vi "Waveplatecontrol_stepscan.vi"() -> ()   [LabVIEW 2015]
uses:
  subvi/Newport ESP301/Newport ESP301.lvlib
  <vilib>/DAQmx/create/channels.llb/DAQmx Create Channel (AO-Voltage-Basic).vi
  <vilib>/DAQmx/write.llb/DAQmx Write (Analog DBL 1Chan 1Samp).vi
panel:
  in  "p1 [deg] 3":dbl
  in  "p1 [deg] 2":dbl
  in  "Numeric":i32=10
  in  "Stepsize":dbl
  in  "ms2wait":u32
  in  "Boolean":bool
  out "a":waveform(dbl)(graph)={"t0"=timestamp(3620209335.8073797 s since 1904-01-01), "dt"=1.0, "Y"=[nan]}
  out "Waveform Chart":dbl(graph)=5.25341140860948
  out "x*y":dbl=nan
  in  "physical channels":tag="Dev3/ao1"
  out "DAC error":errorcluster
  out "ESP error":errorcluster={"status"=TRUE, "code"=-1073807343, "source"="VISA Open in Newport ESP301.lvlib:Initialize.vi->main002.vi"}
  out "run?":bool
  in  "set_vel":bool
  in  "velocity [fs/s]":dbl=667.128190396304
  in  "vel_mm":dbl caption="velocity [deg/s]"
  out "meas. velocity":dbl=nan
  in  "stop":bool
  out "output voltage":dbl=nan
  in  "start":bool
  in  "go2p1":bool
  out "position [deg]":dbl=nan
  in  "p2 [deg]":dbl=2.0
  in  "p1 [deg]":dbl
  in  "interpolate output":bool
  in  "Delta2 [deg]":dbl=6671.281903963041
  in  "Delta1 [deg]":dbl=-6671.281903963041
  in  "Reference [deg]":dbl=1.0
  in  "Axis (1)":i32=2 min=1 max=3
  in  "Serial Link (RS232)":enum16{"RS232", "USB"}(ring)
  in  "VISA resource name":refnum<visa-resource-name>="COM9"
  in  "main_close":bool
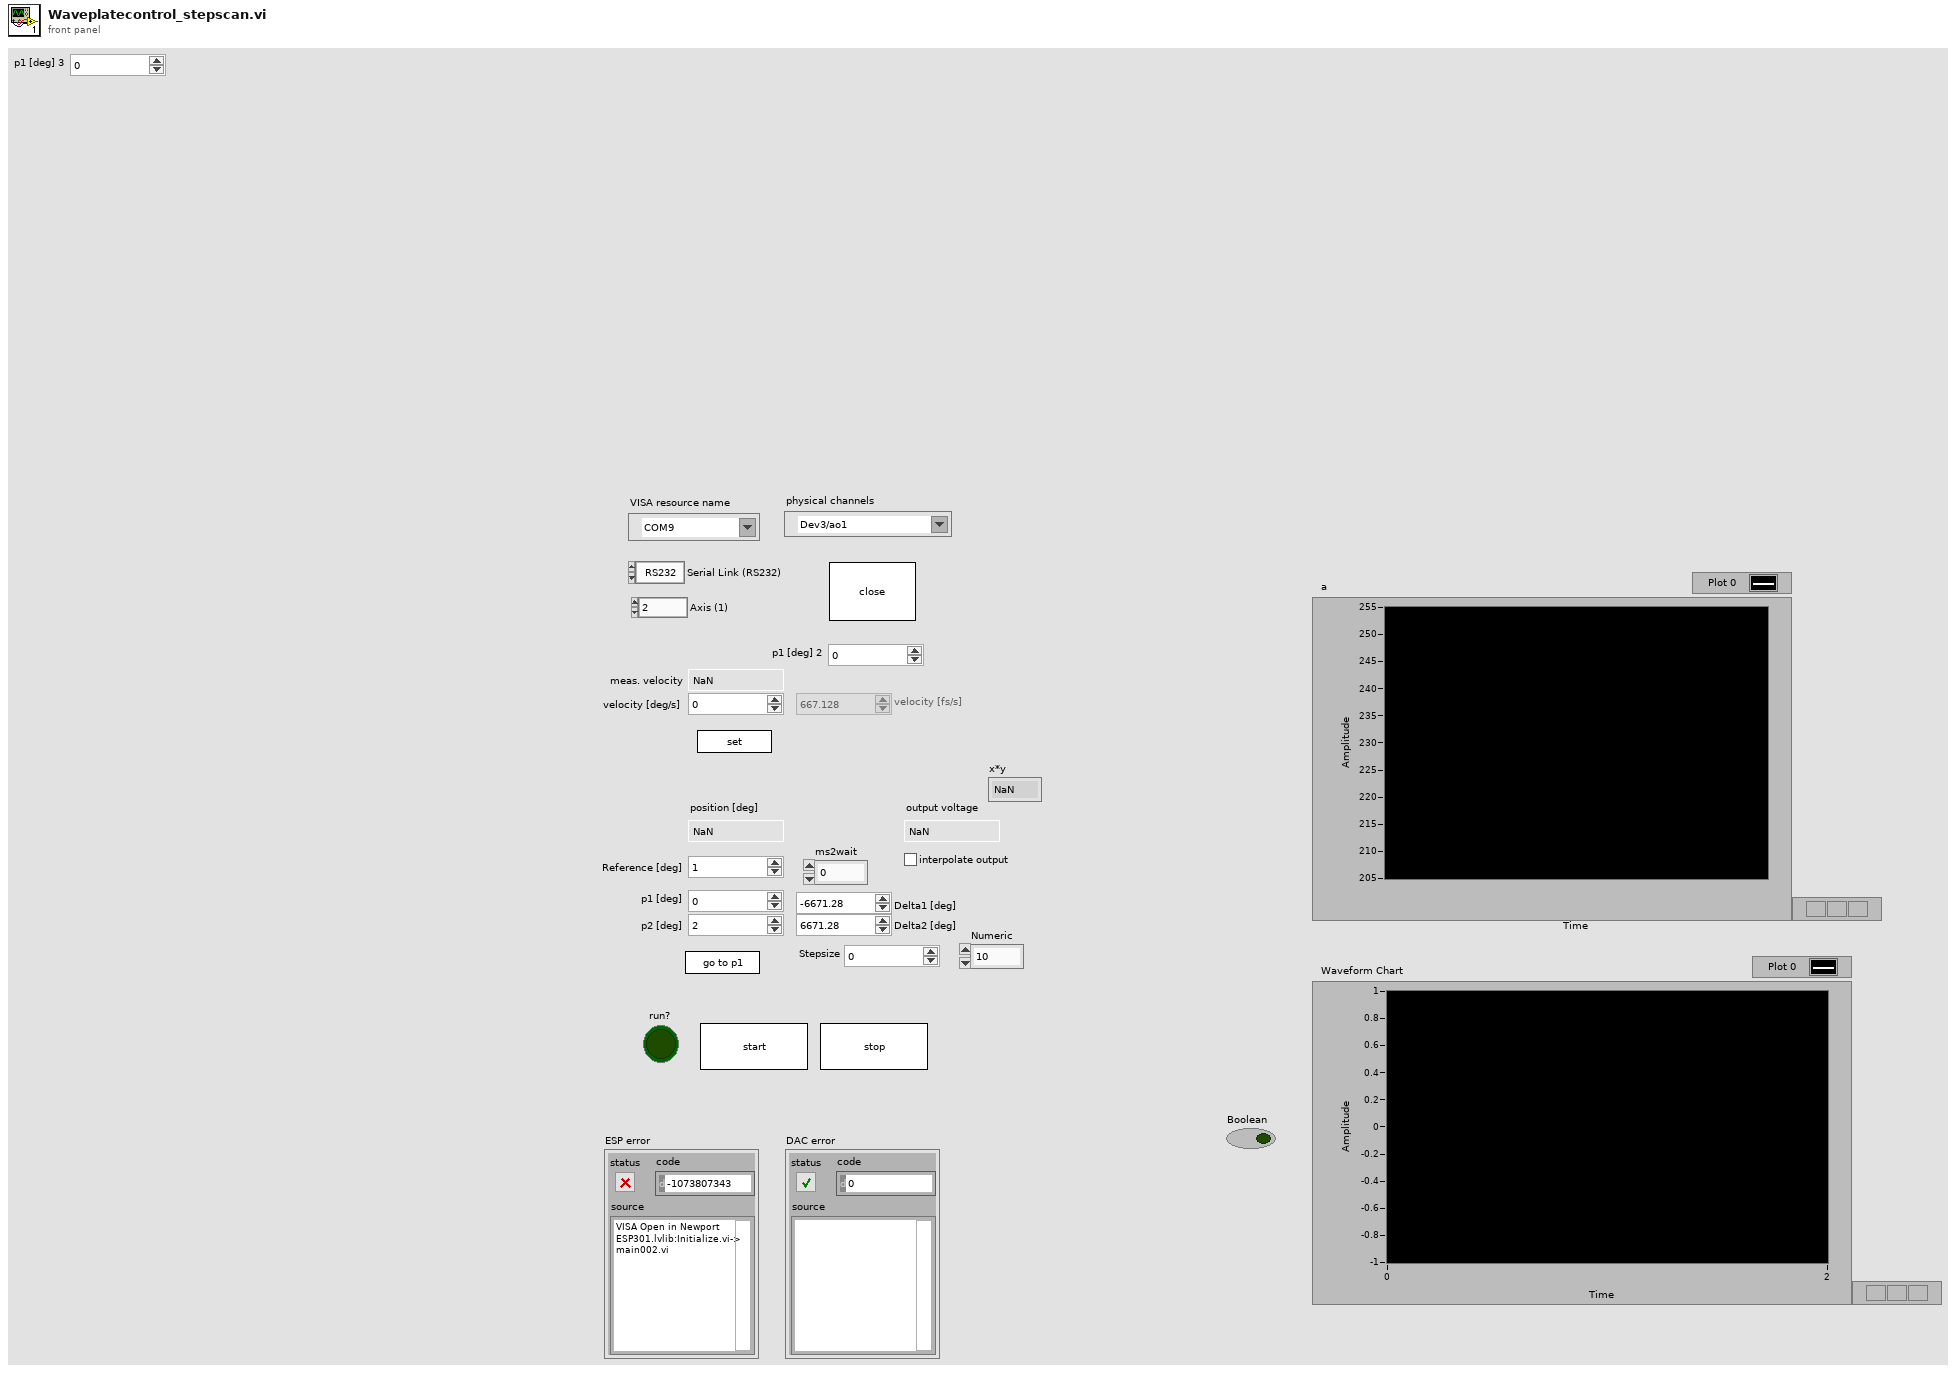
[diagram p1: front panel]
types:
  T1 = cluster{"dev1_data":refnum<queue>, "dev2_data":refnum<queue>}
  T2 = cluster{"dev1_cmd":refnum<queue>, "dev2_cmd":refnum<queue>}
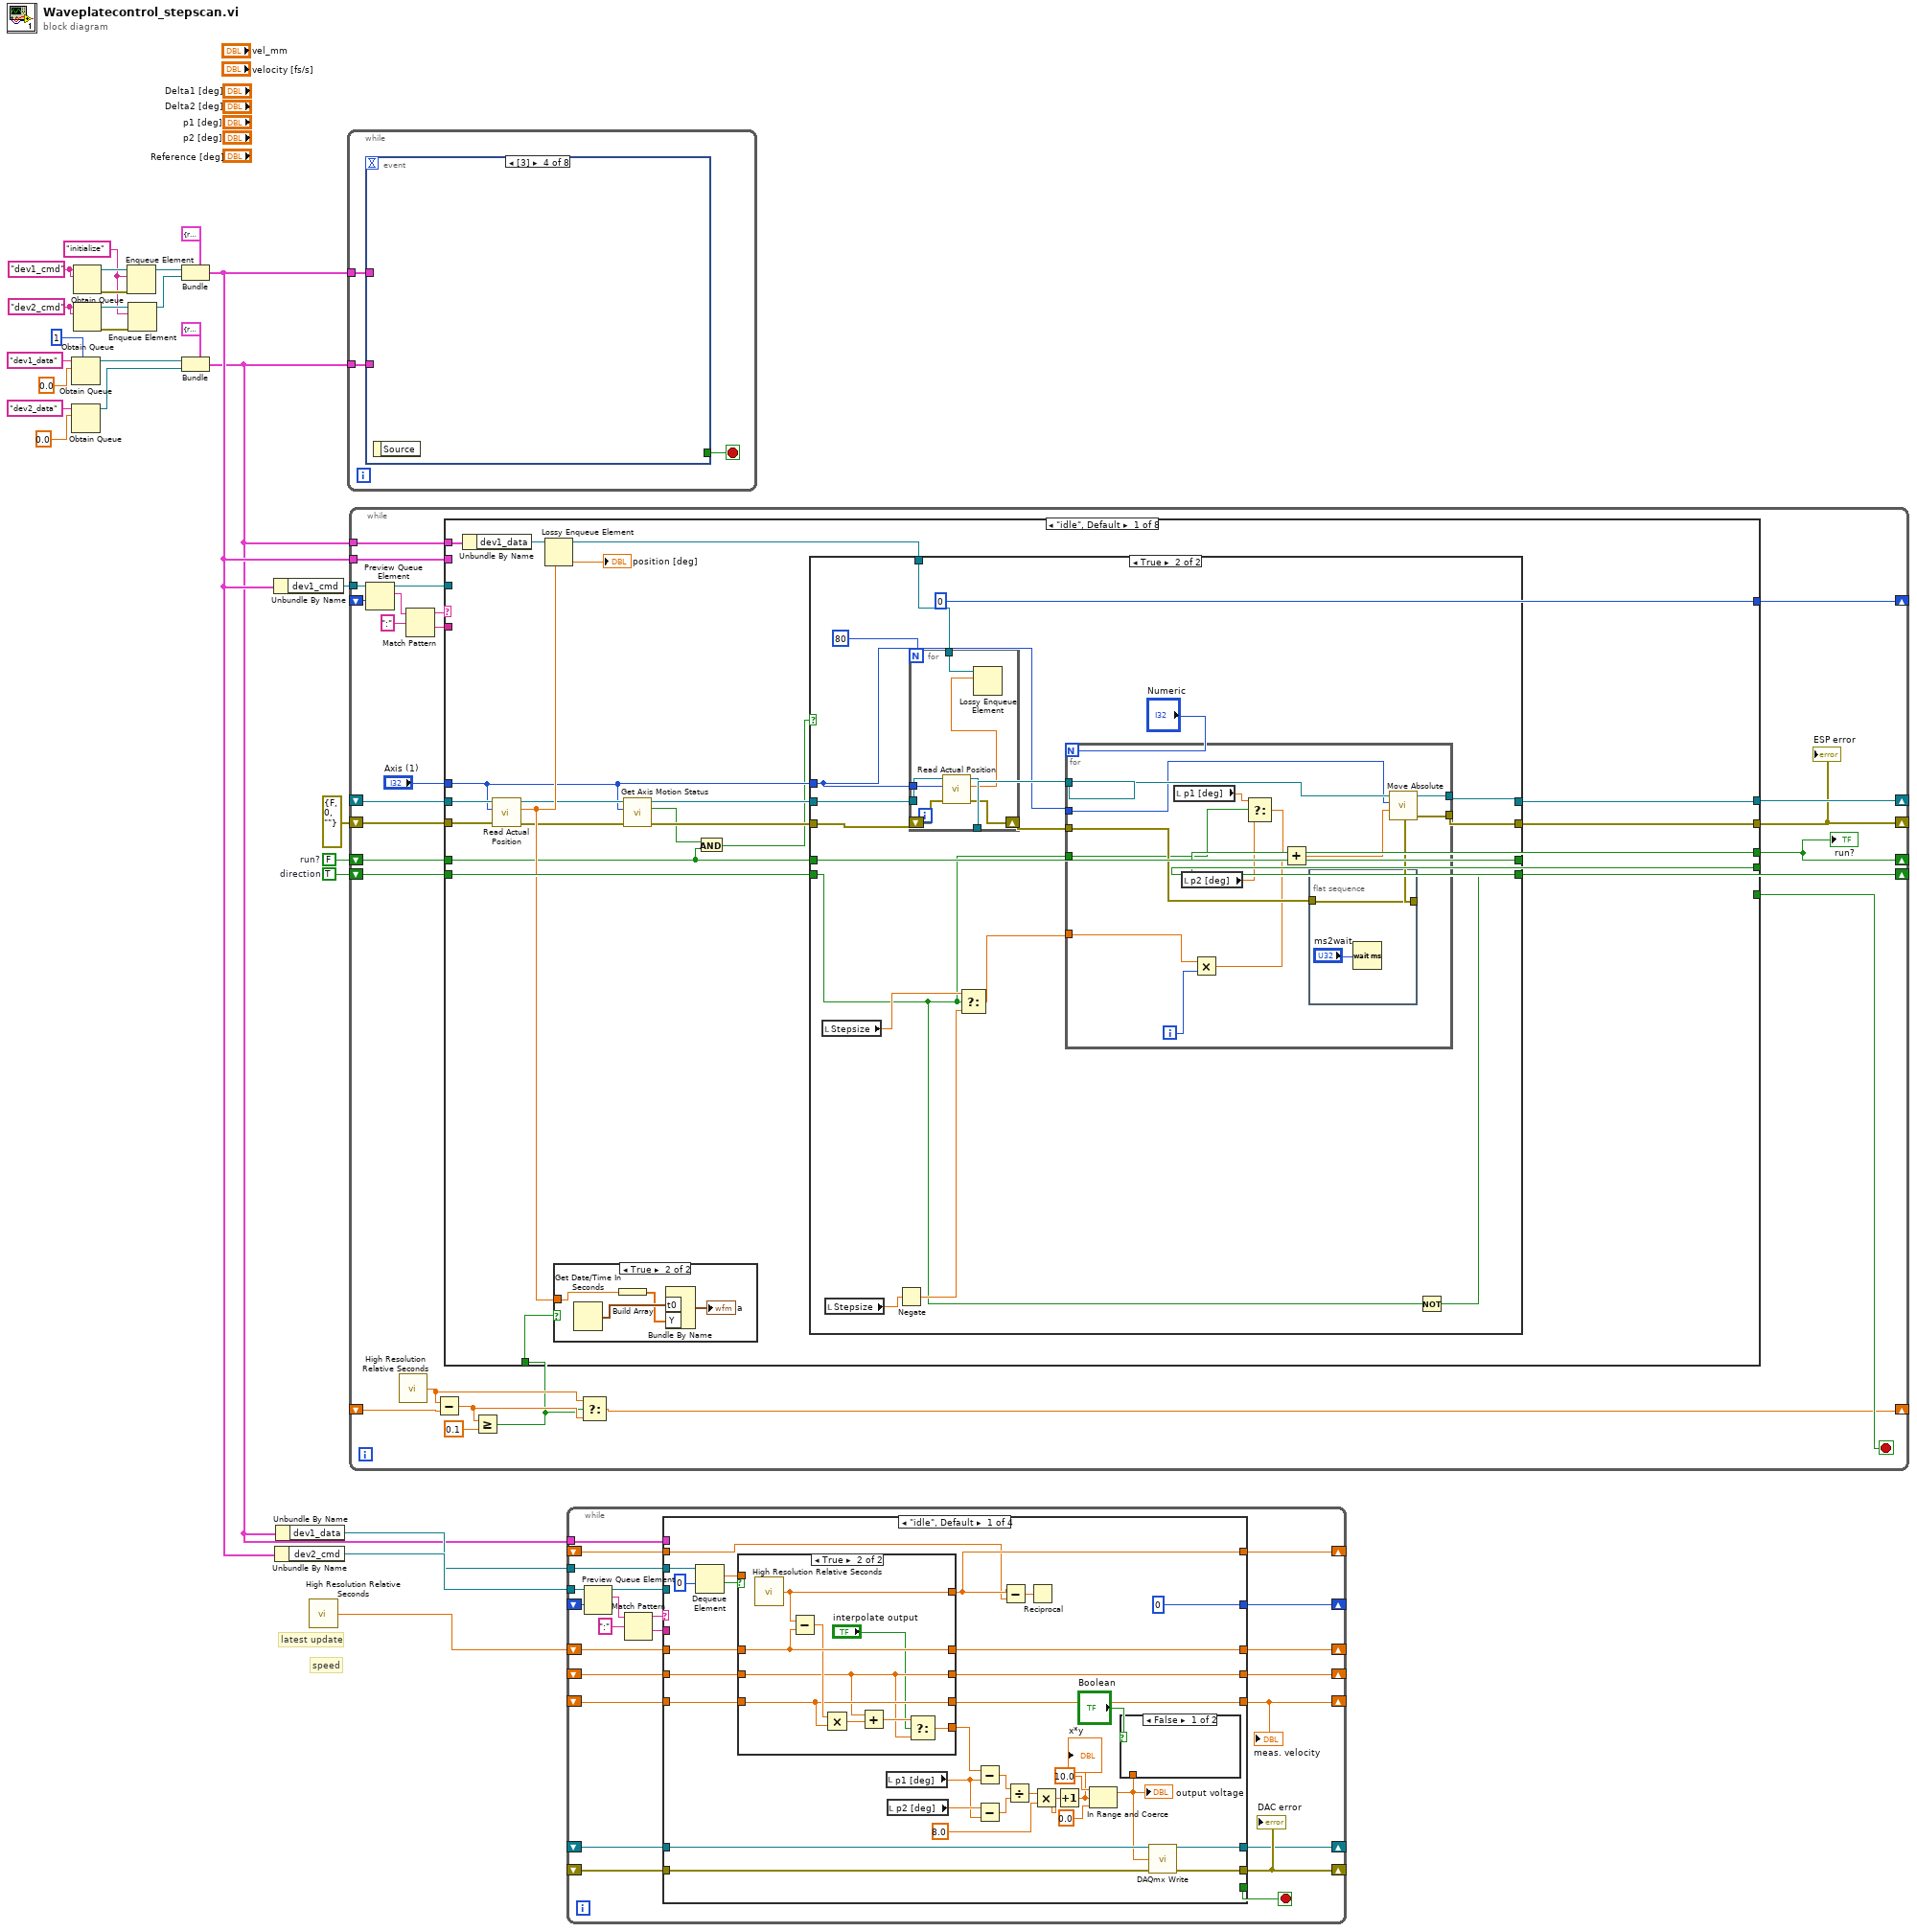
[diagram p0: block diagram]
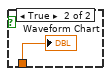
[diagram p2: hidden frame]
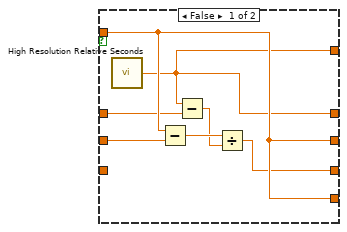
[diagram p3: hidden frame]
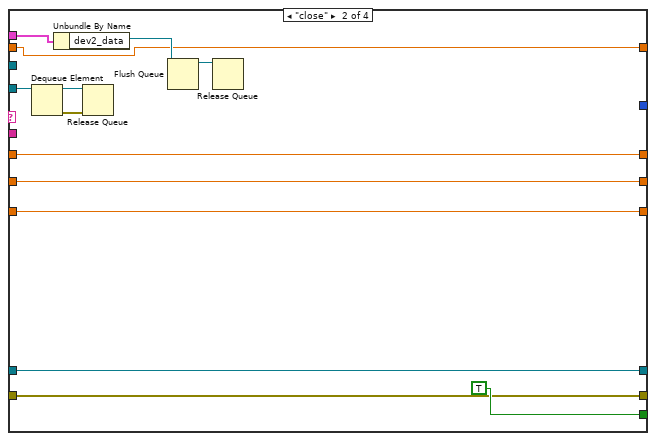
[diagram p4: hidden frame]
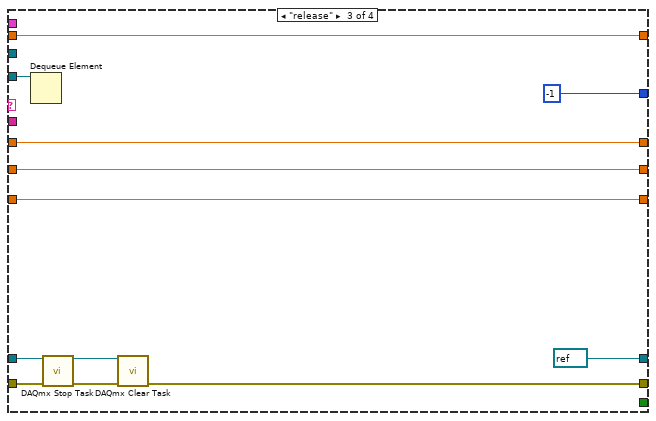
[diagram p5: hidden frame]
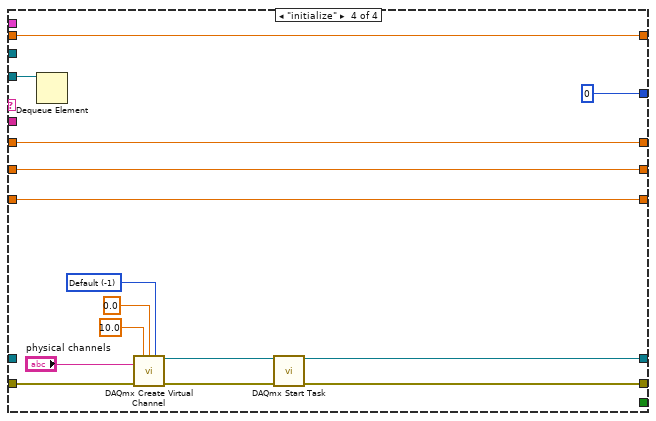
[diagram p6: hidden frame]
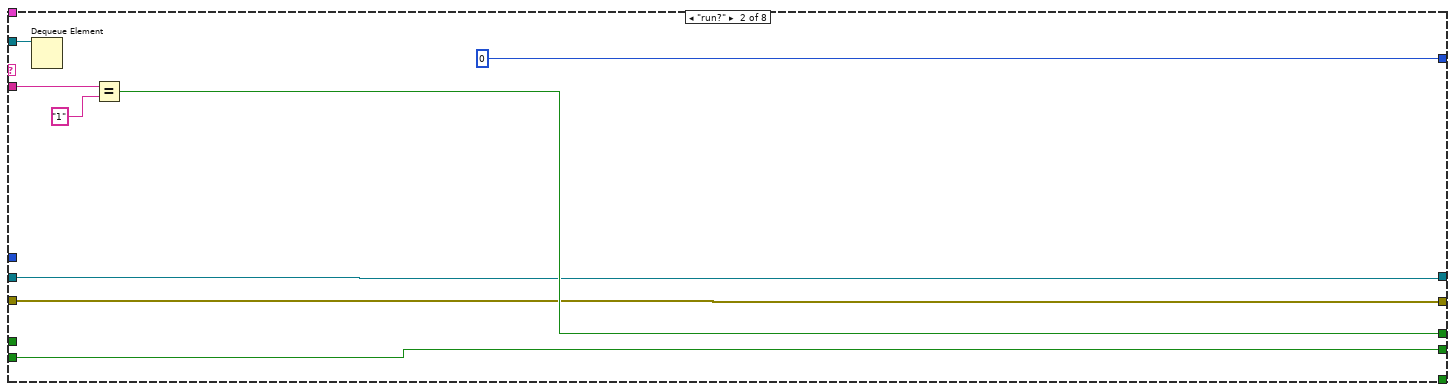
[diagram p9: hidden frame]
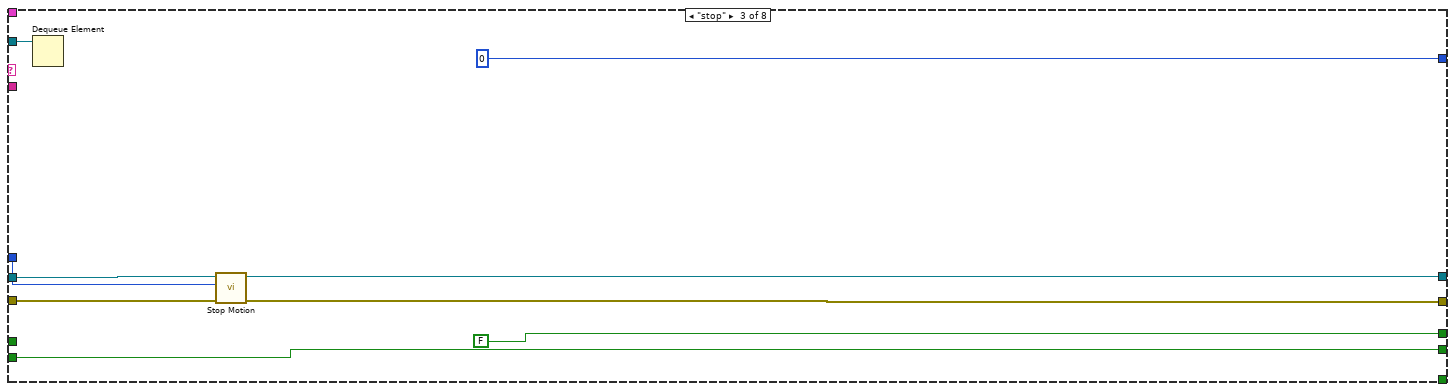
[diagram p10: hidden frame]
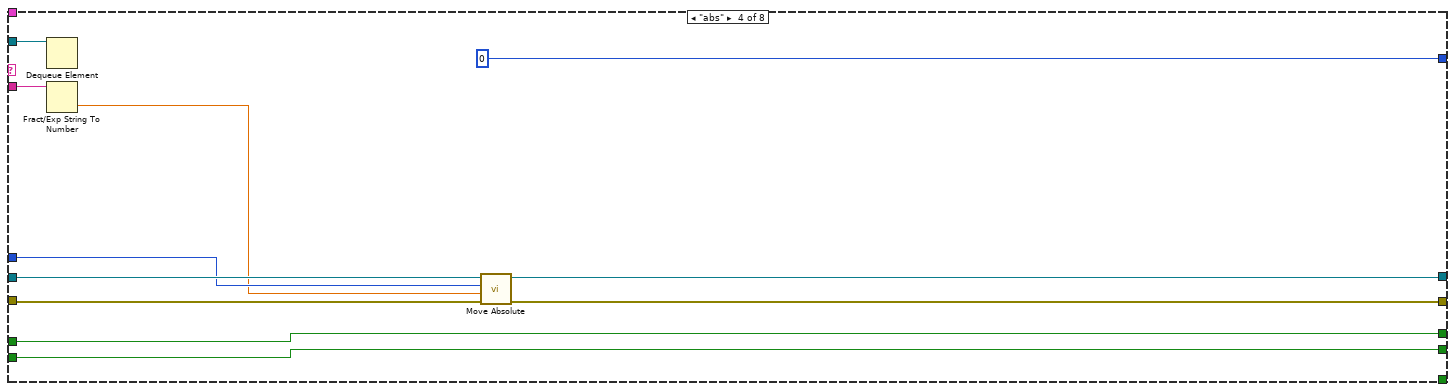
[diagram p11: hidden frame]
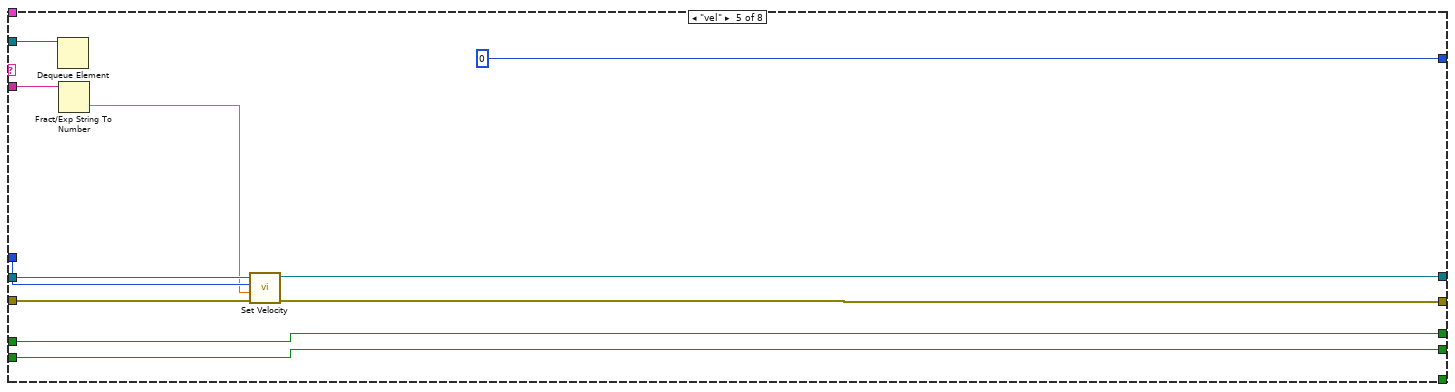
[diagram p12: hidden frame]
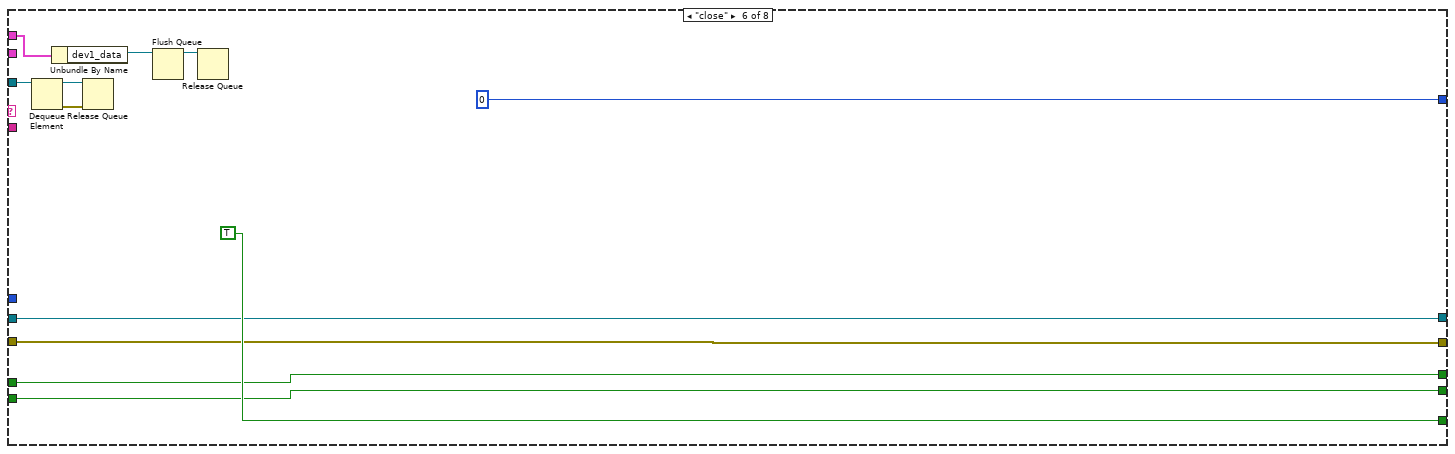
[diagram p13: hidden frame]
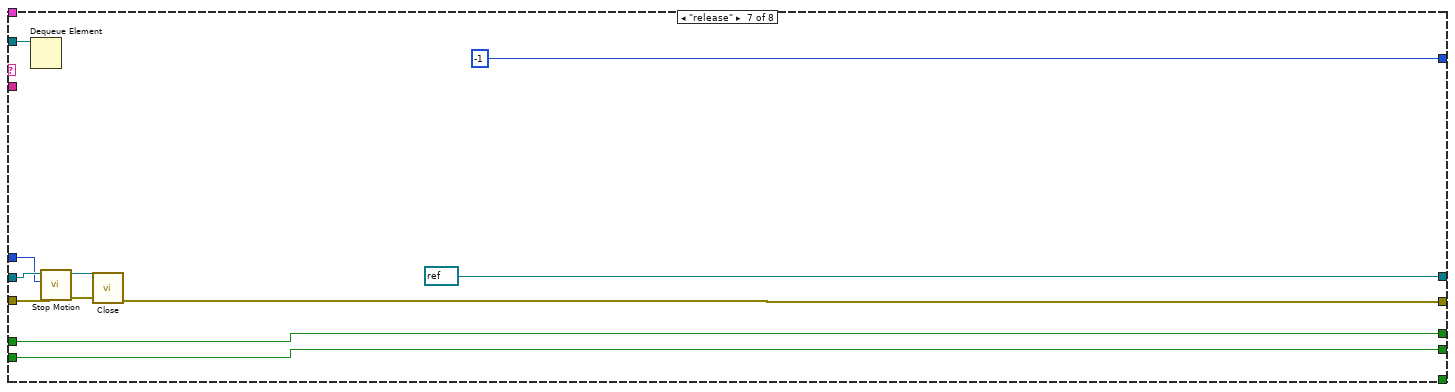
[diagram p14: hidden frame]
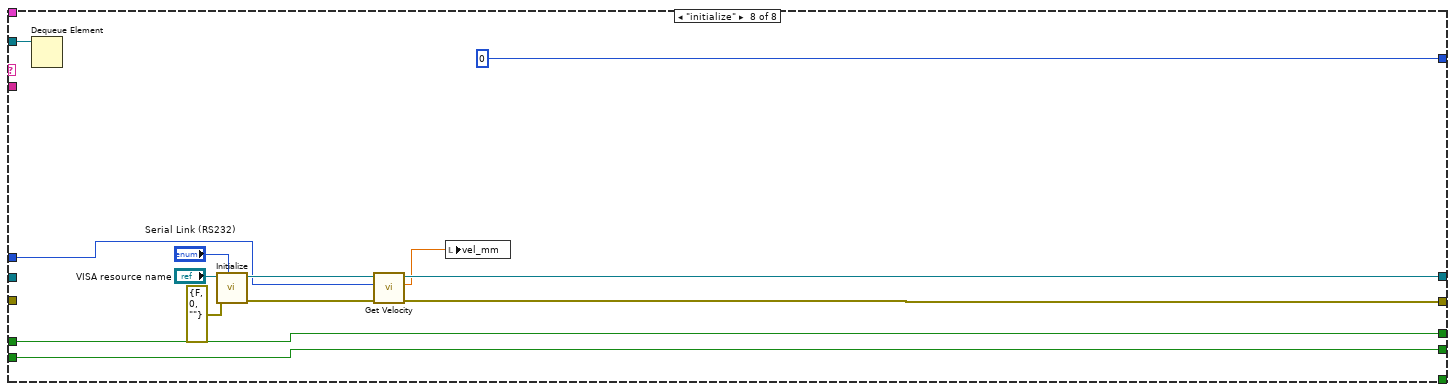
[diagram p15: hidden frame]
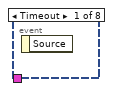
[diagram p16: hidden frame]
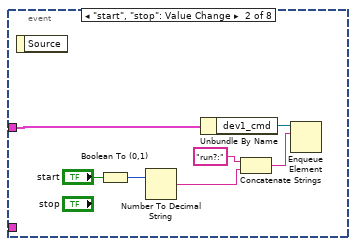
[diagram p17: hidden frame]
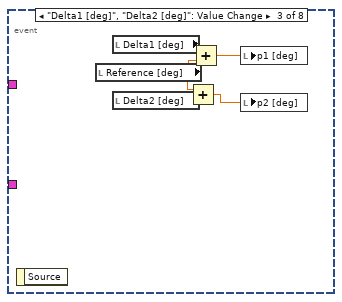
[diagram p18: hidden frame]
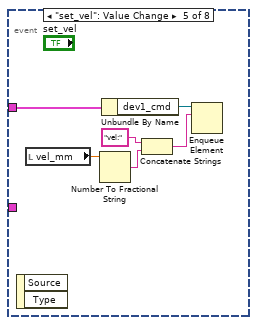
[diagram p19: hidden frame]
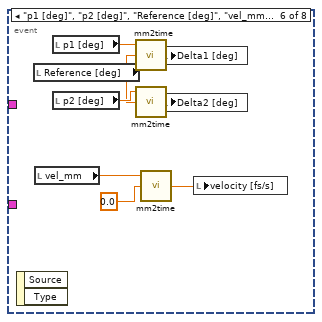
[diagram p20: hidden frame]
diagram:
  w1 = TRUE  # direction
  w4 = FALSE  # run?
  w15 = "dev2_cmd" ("name (unnamed)")
  w21 = "initialize" ("element")
  w16 = "dev1_cmd" ("name (unnamed)")
  # "speed"
  # "latest update"
  n1 = Obtain Queue(max queue size (-1, unlimited)=1, name (unnamed)="dev1_data", element data type=0.0) -> (queue out=w12:refnum<queue>)  [unwired: 2 in, 2 out]
  n2 = Obtain Queue(name (unnamed)="dev2_data", element data type=0.0) -> (queue out=w11:refnum<queue>)  [unwired: 3 in, 2 out]
  n3 = Obtain Queue(name (unnamed)=w16, element data type=w16) -> (queue out=w27:refnum<queue>, error out=w26:errorcluster)  [unwired: 3 in, 1 out]
  n4 = Obtain Queue(name (unnamed)=w15, element data type=w15) -> (queue out=w22:refnum<queue>, error out=w23:errorcluster)  [unwired: 3 in, 1 out]
  n5 = Enqueue Element(queue=w27, element=w21, error in (no error)=w26) -> (queue out=w24:refnum<queue>)  [unwired: 1 in, 2 out]
  n6 = Enqueue Element(queue=w22, element=w21, error in (no error)=w23) -> (queue out=w20:refnum<queue>)  [unwired: 1 in, 2 out]
  n7 = Bundle(cluster=T2 {"dev1_cmd"=refnum, "dev2_cmd"=refnum}, "dev1_cmd"=w24, "dev2_cmd"=w20) -> (w8:T2)
  n8 = Bundle(cluster=T1 {"dev1_data"=refnum, "dev2_data"=refnum}, "dev1_data"=w12, "dev2_data"=w11) -> (w2:T1)
  n9 = Unbundle By Name(w8) -> ("dev1_cmd"=w17:refnum<queue>)
  n10 = Unbundle By Name(w8) -> ("dev2_cmd"=w7:refnum<queue>)
  n11 = Unbundle By Name(w2) -> ("dev1_data"=w6:refnum<queue>)
  n12 = call <vilib>:"High Resolution Relative Seconds.vi"() -> ("relative seconds"=w5:dbl)
  n13 = while {
    tunnel: w8 -> [w30]
    tunnel: w2 -> [w29]
    stop <- w28 stop-if-true
    n14 = event shown="[3]" {
      selector: _ -> [_ _ _ _ _ _ _ _]
      dyn-events: _ -> [_ _ _ _ _ _ _ _]
      timeout: _ -> [_ _ _ _ _ _ _ _]
      tunnel: w30 -> [_ w34 _ _ w44 _ w62 w65]
      tunnel: w29 -> [_ _ _ _ _ _ _ _]
      tunnel: [_ _ _ _ _ _ _ TRUE] -> w28
      event Timeout {
        n15 = event-data() -> ()  [unwired: 1 in, 1 out]
      }
      event "start", "stop": Value Change {
        n16 = event-data() -> ()  [unwired: 1 in, 1 out]
        n17 = Boolean To (0,1)(Boolean="start") -> (0, 1=w32:i16)
        n18 = Number To Decimal String(number=w32) -> (decimal integer string=w31:string)  [unwired: 1 in]
        n19 = Unbundle By Name(w34) -> ("dev1_cmd"=w37:refnum<queue>)
        n20 = Concatenate Strings("run?:" ("string"), w31) -> (w36:string)
        n21 = Enqueue Element(queue=w37, element=w36) -> ()  [unwired: 2 in, 3 out]
      }
      event "Delta1 [deg]", "Delta2 [deg]": Value Change {
        n22 = event-data() -> ()  [unwired: 1 in, 1 out]
        n23 = local read "Reference [deg]"() -> (w40:dbl)
        n24 = local read "Delta1 [deg]"() -> (w42:dbl)
        n25 = local read "Delta2 [deg]"() -> (w41:dbl)
        n26 = Add(x=w40, y=w41) -> (x+y=w38:dbl)
        n27 = Add(x=w42, y=w40) -> (x+y=w39:dbl)
        n28 = local write "p1 [deg]"(w39) -> ()
        n29 = local write "p2 [deg]"(w38) -> ()
      }
      event #3 (no event record) {
        n30 = event-data() -> ()  [unwired: 1 in, 1 out]
        n31 = local read "p1 [deg] 3"() -> ()  [unwired: 1 out]
      }
      event "set_vel": Value Change {
        n32 = event-data() -> ()  [unwired: 1 in, 2 out]
        n33 = local read "vel_mm"() -> (w43:dbl)
        n34 = Number To Fractional String(number=w43) -> (F-format string=w47:string)  [unwired: 3 in]
        n35 = Unbundle By Name(w44) -> ("dev1_cmd"=w48:refnum<queue>)
        n36 = Concatenate Strings("vel:" ("string"), w47) -> (w46:string)
        n37 = Enqueue Element(queue=w48, element=w46) -> ()  [unwired: 2 in, 3 out]
      }
      event "p1 [deg]", "p2 [deg]", "Reference [deg]", "vel_mm": Value Change {
        n38 = event-data() -> ()  [unwired: 1 in, 2 out]
        n39 = local read "Reference [deg]"() -> (w54:dbl)
        n40 = local read "vel_mm"() -> (w51:dbl)
        n41 = local read "p1 [deg]"() -> (w55:dbl)
        n42 = local read "p2 [deg]"() -> (w56:dbl)
        n43 = call "mm2time.vi"("Offset (mm)"=w54, "distance (mm)"=w55) -> ("time in fs"=w52:dbl)  [unwired: 1 in]
        n44 = call "mm2time.vi"("Offset (mm)"=w54, "distance (mm)"=w56) -> ("time in fs"=w53:dbl)  [unwired: 1 in]
        n45 = call "mm2time.vi"("Offset (mm)"=0.0, "distance (mm)"=w51) -> ("time in fs"=w50:dbl)  [unwired: 1 in]
        n46 = local write "Delta1 [deg]"(w52) -> ()
        n47 = local write "Delta2 [deg]"(w53) -> ()
        n48 = local write "velocity [fs/s]"(w50) -> ()
      }
      event "go2p1": Value Change {
        n49 = event-data() -> ()  [unwired: 1 in, 2 out]
        n50 = local read "p1 [deg]"() -> (w57:dbl)
        n51 = Number To Fractional String(number=w57) -> (F-format string=w60:string)  [unwired: 3 in]
        n52 = Unbundle By Name(w62) -> ("dev1_cmd"=w61:refnum<queue>)
        n53 = Concatenate Strings("abs:" ("string"), w60) -> (w58:string)
        n54 = Enqueue Element(queue=w61, element=w58) -> ()  [unwired: 2 in, 3 out]
      }
      event "main_close": Value Change {
        n55 = event-data() -> ()  [unwired: 1 in, 1 out]
        n56 = Cluster To Array(cluster=w65) -> (array=w64:refnum<queue>[])
        n57 = for {
          tunnel: w64 -> [w70] mode=indexing
          n58 = Flush Queue(queue=w70) -> (queue out=w66:refnum<queue>)  [unwired: 1 in, 2 out]
          n59 = Enqueue Element(queue=w66, element="release") -> (queue out=w68:refnum<queue>)  [unwired: 2 in, 2 out]
          n60 = Enqueue Element(queue=w68, element="close") -> ()  [unwired: 2 in, 3 out]
        }
      }
    }
  }
  n61 = while {
    tunnel: w8 -> [w91]
    tunnel: w17 -> [w96]
    tunnel: w2 -> [w88]
    shift-right: [w86] -> _
    shift-left: _ -> [w87]
    shift-right: [w85] -> _
    shift-left: _ -> [w82]
    shift-right: [w84] -> _
    shift-left: errorcluster {"status"=FALSE, "code"=0, "source"=""} ("error out") -> [w83]
    shift-right: [w79] -> _
    shift-left: w4 -> [w80]
    shift-right: [w77] -> _
    shift-left: w1 -> [w78]
    shift-right: [w71] -> _
    shift-left: _ -> [w76]
    stop <- w89 stop-if-true
    n62 = Preview Queue Element(queue=w96, timeout in ms (-1)=w87) -> (queue out=w90:refnum<queue>, element=w95:string)  [unwired: 1 in, 2 out]
    n63 = call <vilib>:"High Resolution Relative Seconds.vi"() -> ("relative seconds"=w73:dbl)
    n64 = Match Pattern(string=w95, regular expression=":") -> (before substring=w93:string, after substring=w92:string)  [unwired: 1 in, 2 out]
    n65 = Subtract(x=w73, y=w76) -> (x-y=w74:dbl)
    n66 = Greater Or Equal?(x=w74, y=0.1) -> (x >= y?=w72:bool)
    n67 = case shown="\"idle\", Default" w93 {
      tunnel: w92 -> [_ w173 _ w192 w199 _ _ _]
      tunnel: w91 -> [_ _ _ _ _ _ _ _]
      tunnel: w90 -> [_ w171 w175 w193 w197 w216 w226 w236]
      tunnel: [_ _ _ _ _ TRUE _ _] -> w89
      tunnel: w88 -> [w116 _ _ _ _ w208 _ _]
      tunnel: [0 0 0 0 0 0 -1 0] -> w86
      tunnel: [w114 w166 w180 w189 w204 w212 refnum<visa-resource-name> refnum ("VISA resource name out") w232] -> w85
      tunnel: [w113 w167 w179 w188 w203 w211 w225 w231] -> w84
      tunnel: w83 -> [w111 w167 w181 w190 w202 w211 w221 _]
      tunnel: w82 -> [w112 w166 w182 w191 w201 w212 w218 _]
      tunnel: "Axis (1)" -> [w100 _ w178 w187 w200 _ w217 w233]
      tunnel: w80 -> [w98 _ _ w184 w195 w209 w223 w237]
      tunnel: [w108 w169 FALSE ("run?") w184 w195 w209 w223 w237] -> w79
      tunnel: w78 -> [w109 w168 w174 w183 w194 w205 w222 w228]
      tunnel: [w110 w168 w174 w183 w194 w205 w222 w228] -> w77
      tunnel: w72 -> [w107 _ _ _ _ _ _ _]
      frame "idle", Default {
        n68 = Unbundle By Name(w116) -> ("dev1_data"=w115:refnum<queue>)
        n69 = call "Read Actual Position.vi"("error in (no error)"=w111, "Axis (1)"=w100, "VISA resource name"=w112) -> ("error out"=w103:errorcluster, "Position (units)"=w105:dbl, "VISA resource name out"=w104:refnum<visa-resource-name>)  [unwired: 2 in]
        "position [deg]" <- w105
        n70 = Lossy Enqueue Element(queue=w115, element=w105) -> (queue out=w106:refnum<queue>)  [unwired: 1 in, 3 out]
        n71 = case shown="True" w107 {
          tunnel: w105 -> [_ w121]
          frame False {
          }
          frame True {
            n72 = Get Date/Time In Seconds() -> (seconds since 1Jan1904=w120:timestamp)
            n73 = Build Array(w121) -> (w119:dbl[])
            n74 = Bundle By Name("t0"=w120, "Y"=w119) -> (→"a":waveform(dbl))  [unwired: 1 in]
          }
        }
        n75 = call "Get Axis Motion Status.vi"("error in (no error)"=w103, "Axis (1)"=w100, "VISA resource name"=w104) -> ("error out"=w101:errorcluster, "Motion Done"=w99:bool, "VISA resource name out"=w102:refnum<visa-resource-name>)  [unwired: 2 in]
        n76 = And(x=w99, y=w98) -> (x .and. y?=w97:bool)
        n77 = case shown="True" w97 {
          tunnel: w102 -> [w125 w138]
          tunnel: w101 -> [w124 w139]
          tunnel: [w125 w134] -> w114
          tunnel: [w124 w135] -> w113
          tunnel: w100 -> [_ w132]
          tunnel: [w123 w137] -> w110
          tunnel: w109 -> [w123 w126]
          tunnel: w98 -> [w122 w142]
          tunnel: [w122 w142] -> w108
          tunnel: w106 -> [_ w141]
          frame False {
          }
          frame True {
            n78 = local read "Stepsize"() -> (w136:dbl)
            n79 = local read "Stepsize"() -> (w130:dbl)
            n80 = Negate(x=w130) -> (-x=w129:dbl)
            n81 = for {
              N: 80 -> [_]
              tunnel: w138 -> [w165]
              tunnel: [w164] -> w133
              shift-right: [w159] -> w131
              shift-left: w139 -> [w163]
              tunnel: w132 -> [w162]
              tunnel: w141 -> [w161]
              n82 = call "Read Actual Position.vi"("error in (no error)"=w163, "Axis (1)"=w162, "VISA resource name"=w165) -> ("error out"=w159:errorcluster, "Position (units)"=w160:dbl, "VISA resource name out"=w164:refnum<visa-resource-name>)  [unwired: 2 in]
              n83 = Lossy Enqueue Element(queue=w161, element=w160) -> ()  [unwired: 1 in, 4 out]
            }
            n84 = Select(t=w136, s=w126, f=w129) -> (s? t:f=w128:dbl)
            n85 = for {
              N: "Numeric" -> [_]
              tunnel: [w156] -> w135
              tunnel: [w155] -> w134
              tunnel: w131 -> [w152]
              tunnel: w133 -> [w154]
              tunnel: w132 -> [w153]
              tunnel: w128 -> [w149]
              tunnel: w126 -> [w144]
              i -> [w150]
              n86 = local read "p1 [deg]"() -> (w146:dbl)
              n87 = local read "p2 [deg]"() -> (w143:dbl)
              n88 = Multiply(x=w149, y=w150) -> (x*y=w148:dbl)
              n89 = Select(t=w146, s=w144, f=w143) -> (s? t:f=w145:dbl)
              n90 = Add(x=w145, y=w148) -> (x+y=w147:dbl)
              n91 = flat-sequence {
                tunnel: w152 -> [w158]
                tunnel: [w158] -> w151
                frame #0 {
                  n92 = Wait (ms)(milliseconds to wait="ms2wait") -> ()  [unwired: 1 out]
                }
              }
              n93 = call "Move Absolute.vi"("error in (no error)"=w151, "Position (0 units)"=w147, "Axis (1)"=w153, "VISA resource name"=w154) -> ("error out"=w156:errorcluster, "VISA resource name out"=w155:refnum<visa-resource-name>)  [unwired: 2 in]
              n94 = local read "p1 [deg] 2"() -> ()  [unwired: 1 out]
            }
            n95 = Not(x=w126) -> (.not. x?=w137:bool)
          }
        }
      }
      frame "run?" {
        n96 = Dequeue Element(queue=w171) -> ()  [unwired: 2 in, 4 out]
        n97 = Equal?(x=w173, y="1") -> (x = y?=w169:bool)
      }
      frame "stop" {
        n98 = Dequeue Element(queue=w175) -> ()  [unwired: 2 in, 4 out]
        n99 = call "Stop Motion.vi"("error in (no error)"=w181, "Axis (1)"=w178, "VISA resource name"=w182) -> ("error out"=w179:errorcluster, "VISA resource name out"=w180:refnum<visa-resource-name>)  [unwired: 3 in]
      }
      frame "abs" {
        n100 = Dequeue Element(queue=w193) -> ()  [unwired: 2 in, 4 out]
        n101 = Fract/Exp String To Number(string=w192) -> (number=w186:dbl)  [unwired: 3 in, 1 out]
        n102 = call "Move Absolute.vi"("error in (no error)"=w190, "Position (0 units)"=w186, "Axis (1)"=w187, "VISA resource name"=w191) -> ("error out"=w188:errorcluster, "VISA resource name out"=w189:refnum<visa-resource-name>)  [unwired: 2 in]
      }
      frame "vel" {
        n103 = Dequeue Element(queue=w197) -> ()  [unwired: 2 in, 4 out]
        n104 = Fract/Exp String To Number(string=w199) -> (number=w198:dbl)  [unwired: 3 in, 1 out]
        n105 = call "Set Velocity.vi"("error in (no error)"=w202, "Velocity (units/s)"=w198, "Axis (1)"=w200, "VISA resource name"=w201) -> ("error out"=w203:errorcluster, "VISA resource name out"=w204:refnum<visa-resource-name>)  [unwired: 2 in]
      }
      frame "close" {
        n106 = Dequeue Element(queue=w216) -> (queue out=w215:refnum<queue>, error out=w214:errorcluster)  [unwired: 2 in, 2 out]
        n107 = Unbundle By Name(w208) -> ("dev1_data"=w206:refnum<queue>)
        n108 = Release Queue(queue=w215, error in (no error)=w214) -> ()  [unwired: 1 in, 3 out]
        n109 = Flush Queue(queue=w206) -> (queue out=w207:refnum<queue>)  [unwired: 1 in, 2 out]
        n110 = Release Queue(queue=w207) -> ()  [unwired: 2 in, 3 out]
      }
      frame "release" {
        n111 = Dequeue Element(queue=w226) -> ()  [unwired: 2 in, 4 out]
        n112 = call "Stop Motion.vi"("error in (no error)"=w221, "Axis (1)"=w217, "VISA resource name"=w218) -> ("error out"=w220:errorcluster, "VISA resource name out"=w219:refnum<visa-resource-name>)  [unwired: 3 in]
        n113 = call "Close.vi"("error in (no error)"=w220, "VISA resource name"=w219) -> ("error out"=w225:errorcluster)  [unwired: 9 in]
      }
      frame "initialize" {
        n114 = Dequeue Element(queue=w236) -> ()  [unwired: 2 in, 4 out]
        n115 = call "Initialize.vi"("VISA resource name"="VISA resource name", "error in (no error)"=errorcluster {"status"=FALSE, "code"=0, "source"=""}, "Serial Link (RS232)"="Serial Link (RS232)") -> ("VISA resource name out"=w235:refnum<visa-resource-name>, "error out"=w234:errorcluster)  [unwired: 6 in]
        n116 = call "Get Velocity.vi"("error in (no error)"=w234, "Axis (1)"=w233, "VISA resource name"=w235) -> ("error out"=w231:errorcluster, "Velocity (units/s)"=w230:dbl, "VISA resource name out"=w232:refnum<visa-resource-name>)  [unwired: 2 in]
        n117 = local write "vel_mm"(w230) -> ()
      }
    }
    "run?" <- w79
    "ESP error" <- w84
    n118 = Select(t=w73, s=w72, f=w74) -> (s? t:f=w71:dbl)
  }
  n119 = while {
    shift-right: [w256] -> _
    shift-left: _ -> [w257]
    shift-right: [w255] -> _
    shift-left: _ -> [w254]
    tunnel: w7 -> [w253]
    shift-right: [w252] -> _
    shift-left: _ -> [w251]
    tunnel: w6 -> [w250]
    shift-right: [w249] -> _
    shift-left: _ -> [w247]
    shift-right: [w241] -> _
    shift-left: w5 -> [w248]
    shift-right: [w242] -> _
    shift-left: _ -> [w246]
    tunnel: w2 -> [w245]
    shift-right: [w244] -> _
    shift-left: _ -> [w243]
    stop <- w258 stop-if-true
    n120 = Preview Queue Element(queue=w253, timeout in ms (-1)=w257) -> (queue out=w259:refnum<queue>, element=w263:string)  [unwired: 1 in, 2 out]
    n121 = Match Pattern(string=w263, regular expression=":") -> (before substring=w261:string, after substring=w260:string)  [unwired: 1 in, 2 out]
    n122 = case shown="\"idle\", Default" w261 {
      tunnel: w260 -> [_ _ _ _]
      tunnel: w259 -> [_ w324 w335 w343]
      tunnel: [_ TRUE _ _] -> w258
      tunnel: [0 _ -1 0] -> w256
      tunnel: [w290 w320 w334 w344] -> w255
      tunnel: w254 -> [w288 w320 w331 w351]
      tunnel: [w291 w319 refnum<k21> refnum ("task out") w345] -> w252
      tunnel: w251 -> [w289 w319 w332 _]
      tunnel: w250 -> [w292 _ _ _]
      tunnel: [w286 w317 w327 w340] -> w249
      tunnel: [w285 w318 w328 w341] -> w241
      tunnel: w248 -> [w283 w318 w328 w341]
      tunnel: w247 -> [w284 w317 w327 w340]
      tunnel: [w282 w316 w326 w339] -> w242
      tunnel: w246 -> [w281 w316 w326 w339]
      tunnel: w245 -> [_ w313 _ _]
      tunnel: [w270 w312 w325 w337] -> w244
      tunnel: w243 -> [w269 w312 w325 w337]
      frame "idle", Default {
        n123 = Dequeue Element(queue=w292, timeout in ms (-1)=0) -> (element=w287:dbl, timed out?=w271:bool)  [unwired: 1 in, 2 out]
        n124 = case shown="True" w271 {
          tunnel: w287 -> [w302 _]
          tunnel: [w302 w304] -> w280
          tunnel: [w302 w306] -> w286
          tunnel: [w296 w311] -> w285
          tunnel: w284 -> [w301 w306]
          tunnel: w283 -> [w300 w311]
          tunnel: [w297 w308] -> w282
          tunnel: w281 -> [_ w308]
          tunnel: [w296 w303] -> w270
          frame False {
            n125 = call <vilib>:"High Resolution Relative Seconds.vi"() -> ("relative seconds"=w296:dbl)
            n126 = Subtract(x=w302, y=w301) -> (x-y=w299:dbl)
            n127 = Subtract(x=w296, y=w300) -> (x-y=w298:dbl)
            n128 = Divide(x=w299, y=w298) -> (x/y=w297:dbl)
          }
          frame True {
            n129 = call <vilib>:"High Resolution Relative Seconds.vi"() -> ("relative seconds"=w303:dbl)
            n130 = Subtract(x=w303, y=w311) -> (x-y=w310:dbl)
            n131 = Multiply(x=w310, y=w308) -> (x*y=w309:dbl)
            n132 = Add(x=w306, y=w309) -> (x+y=w307:dbl)
            n133 = Select(t=w307, s="interpolate output", f=w306) -> (s? t:f=w304:dbl)
          }
        }
        n134 = local read "p1 [deg]"() -> (w278:dbl)
        n135 = local read "p2 [deg]"() -> (w279:dbl)
        n136 = Subtract(x=w280, y=w278) -> (x-y=w277:dbl)
        n137 = Subtract(x=w279, y=w278) -> (x-y=w276:dbl)
        n138 = Subtract(x=w270, y=w269) -> (x-y=w268:dbl)
        n139 = Divide(x=w277, y=w276) -> (x/y=w275:dbl)
        n140 = Reciprocal(x=w268) -> ()  [unwired: 1 out]
        n141 = Multiply(x=w275, y=8.0) -> (x*y=w266:dbl)
        n142 = Increment(x=w266) -> (x+1=w265:dbl)
        "x*y" <- w265
        n143 = In Range and Coerce(upper limit=10.0, x=w265, lower limit=0.0) -> (coerced(x)=w267:dbl)  [unwired: 1 out]
        "output voltage" <- w267
        n144 = case shown="False" "Boolean" {
          tunnel: w267 -> [_ w295]
          frame False {
          }
          frame True {
            "Waveform Chart" <- w295
          }
        }
        n145 = call-poly <vilib>:"DAQmx Write.vi"("task/channels in"=w289, "data"=w267, "error in"=w288) -> ("task out"=w291:refnum<k21>, "error out"=w290:errorcluster)  [unwired: 10 in, 1 out]
      }
      frame "close" {
        n146 = Dequeue Element(queue=w324) -> (queue out=w323:refnum<queue>, error out=w322:errorcluster)  [unwired: 2 in, 2 out]
        n147 = Unbundle By Name(w313) -> ("dev2_data"=w314:refnum<queue>)
        n148 = Release Queue(queue=w323, error in (no error)=w322) -> ()  [unwired: 1 in, 3 out]
        n149 = Flush Queue(queue=w314) -> (queue out=w315:refnum<queue>)  [unwired: 1 in, 2 out]
        n150 = Release Queue(queue=w315) -> ()  [unwired: 2 in, 3 out]
      }
      frame "release" {
        n151 = Dequeue Element(queue=w335) -> ()  [unwired: 2 in, 4 out]
        n152 = call <vilib>:"DAQmx Stop Task.vi"("task/channels in"=w332, "error in"=w331) -> ("task out"=w330:refnum<k21>, "error out"=w329:errorcluster)  [unwired: 12 in]
        n153 = call <vilib>:"DAQmx Clear Task.vi"("task in"=w330, "error in"=w329) -> ("error out"=w334:errorcluster)  [unwired: 13 in]
      }
      frame "initialize" {
        w348 = -1 items=["Default"=-1, "RSE"=10083, "Differential"=10106, "Pseudodifferential"=12529] ("output terminal configuration")
        n154 = Dequeue Element(queue=w343) -> ()  [unwired: 2 in, 4 out]
        n155 = call-poly <vilib>:"DAQmx Create Virtual Channel.vi"("maximum value"=10.0, "minimum value"=0.0, "output terminal configuration"=w348, "physical channels"="physical channels", "error in"=w351) -> ("task out"=w347:refnum<k21>, "error out"=w346:errorcluster)  [unwired: 9 in]
        n156 = call <vilib>:"DAQmx Start Task.vi"("task/channels in"=w347, "error in"=w346) -> ("task out"=w345:refnum<k21>, "error out"=w344:errorcluster)  [unwired: 12 in]
      }
    }
    "meas. velocity" <- w242
    "DAC error" <- w255
  }
